vi "svc_Set SV Channel Info (variant).vi"(5 "channel description":string, 7 "channel name":string, 8 "error in (no error)":errorcluster, 10 "channel info":T1={"sensor sensitivity"=1000.0, "engineering units"=0, "dB reference"=1.0, "custom label"="EU", "weighting filter"=0, "pregain"=0.0} {"pregain" format="%.2f"; "weighting filter" items=["Linear", "A-weighting", "B-weighting", "C-weighting", "ITU-R 468-4", "Dolby", "CCITT", "C-message", "Wb", "Wc", "Wd", "We", "Wf", "Wh", "Wj", "Wk", "Wm", "AES17 20 kHz lowpass", "AES17 40 kHz lowpass", "AES17 20 kHz highpass", "AES17 40 kHz highpass"]; "dB reference" format="%^.1e"; "engineering units" items=["custom..."=0, "V"=1, "A"=21, "C"=30, "pC"=31, "s"=32, "-"=29, "Pa"=2, "N"=20, "g"=3, "m/s^2"=4, "m/s"=5, "m"=6, "mm/s"=12, "mm"=13, "micron/s"=14, "micron"=15, "in/s^2"=7, "in/s"=8, "in"=9, "mil/s"=10, "mil"=11, "rad/s^2"=16, "rad/s"=17, "rad"=18, "deg/s^2"=26, "deg/s"=27, "deg"=28, "RPM"=22, "cycle/s^2"=23, "Hz"=24, "cycle"=25, "strain"=19]; "sensor sensitivity" format="%#_5f"}, 11 "attributes":variant) -> (0 "error out":errorcluster, 3 "attributes":variant)   [LabVIEW 2017]
uses:
  <vilib>/addons/_NISVFA/_Shared subVIs/Controls/svc_Channel Info.ctl
  <vilib>/addons/_NISVFA/_Shared subVIs/Controls/svc_Engineering Units Text Ring.ctl
  <vilib>/addons/_NISVFA/_Shared subVIs/Controls/svc_Weighting Filter Text Ring.ctl
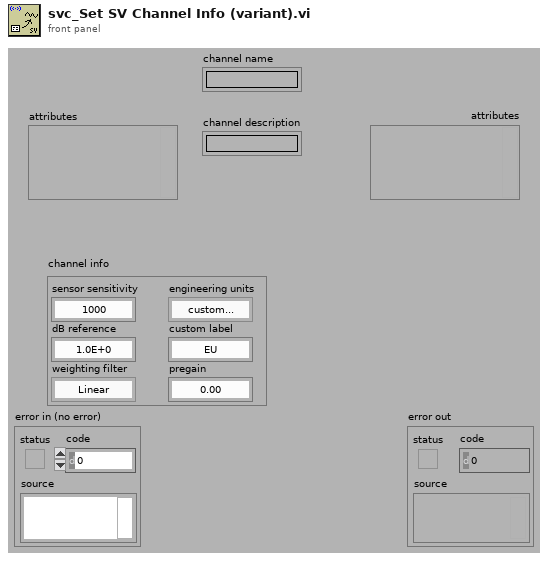
[diagram p1: front panel]
types:
  T1 = typedef "svc_Channel Info.ctl" = cluster{"sensor sensitivity":dbl, "engineering units":T2, "dB reference":dbl, "custom label":string, "weighting filter":T3, "pregain":dbl}
  T2 = typedef "svc_Engineering Units Text Ring.ctl" = u16
  T3 = typedef "svc_Weighting Filter Text Ring.ctl" = u16
  T4 = enum16{"custom...", "V", "Pa", "g", "m/s^2", "m/s", "m", "in/s^2", "in/s", "in", "mil/s", "mil", "mm/s", "mm", "micron/s", "micron", "rad/s^2", "rad/s", "rad", "strain", "N", "A", "rpm", "cycle/s^2", "Hz", "cycle", "deg/s^2", "deg/s", "deg", "Undefined", "C", "pC"}
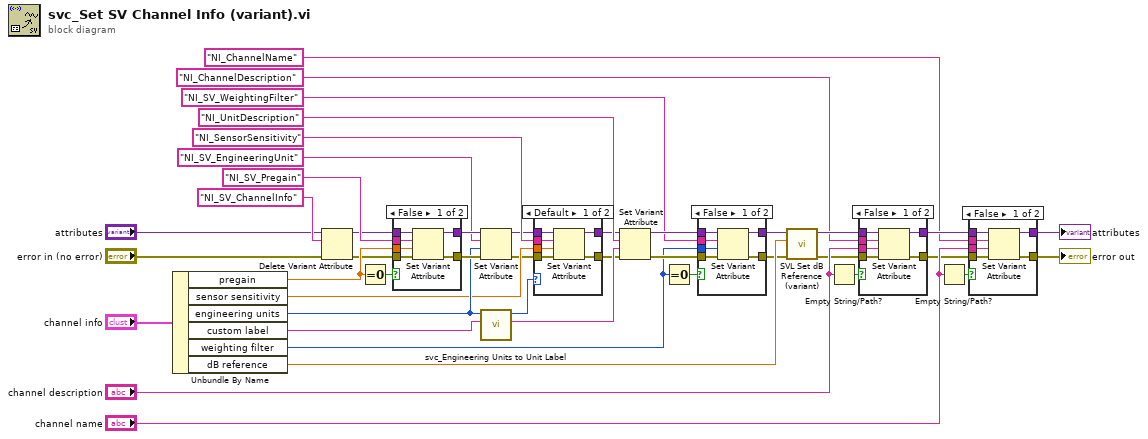
[diagram p0: block diagram]
diagram:
  n1 = Unbundle By Name("channel info") -> ("pregain"=w29:dbl, "sensor sensitivity"=w11:dbl, "engineering units"=w24:T2, "custom label"=w23:string, "weighting filter"=w14:T3, "dB reference"=w20:dbl)
  n2 = Delete Variant Attribute(4:"error in (no error)", 6:"NI_SV_ChannelInfo" ("name"), 7:"attributes") -> (0:w4:errorcluster, 3:w6:variant)  [unwired: 1 out]
  n3 = Equal To 0?(x=w29) -> (x = 0?=w30:bool)
  n4 = case shown="False" w30 {
    tunnel: w6 -> [w49 w51]
    tunnel: [w48 w51] -> w26
    tunnel: [w47 w50] -> w27
    tunnel: w4 -> [w46 w50]
    tunnel: w29 -> [w45 _]
    tunnel: "NI_SV_Pregain" ("name") -> [w44 _]
    frame False {
      n5 = Set Variant Attribute(Variant=w49, name=w44, value=w45, error in=w46) -> (Variant out=w48:variant, error out=w47:errorcluster)  [unwired: 1 out]
    }
    frame True {
    }
  }
  n6 = Set Variant Attribute(Variant=w26, name="NI_SV_EngineeringUnit", value=w24, error in=w27) -> (Variant out=w10:variant, error out=w9:errorcluster)  [unwired: 1 out]
  n7 = call <vilib>:"svc_Engineering Units to Unit Label.vi"("custom label"=w23, "engineering units"=w24) -> ("unit label"=w22:string, "engineering units enum"=w12:T4)  [unwired: 8 in]
  n8 = case shown="Default" w12 {
    tunnel: w10 -> [w57 w59]
    tunnel: [w56 w59] -> w8
    tunnel: [w55 w58] -> w7
    tunnel: w9 -> [w54 w58]
    tunnel: w11 -> [w53 _]
    tunnel: "NI_SensorSensitivity" ("name") -> [w52 _]
    frame Default {
      n9 = Set Variant Attribute(Variant=w57, name=w52, value=w53, error in=w54) -> (Variant out=w56:variant, error out=w55:errorcluster)  [unwired: 1 out]
    }
    frame "V" {
    }
  }
  n10 = Set Variant Attribute(Variant=w8, name="NI_UnitDescription", value=w22, error in=w7) -> (Variant out=w17:variant, error out=w16:errorcluster)  [unwired: 1 out]
  n11 = Equal To 0?(x=w14) -> (x = 0?=w13:bool)
  n12 = case shown="False" w13 {
    tunnel: w17 -> [w65 w67]
    tunnel: [w64 w67] -> w19
    tunnel: [w63 w66] -> w18
    tunnel: w16 -> [w62 w66]
    tunnel: w14 -> [w61 _]
    tunnel: "NI_SV_WeightingFilter" ("name") -> [w60 _]
    frame False {
      n13 = Set Variant Attribute(Variant=w65, name=w60, value=w61, error in=w62) -> (Variant out=w64:variant, error out=w63:errorcluster)  [unwired: 1 out]
    }
    frame True {
    }
  }
  n14 = call <vilib>:"SVL Set dB Reference (variant).vi"("error in (no error)"=w18, "dB reference [EU]"=w20, "attributes in"=w19) -> ("error out"=w36:errorcluster, "attributes out"=w39:variant)  [unwired: 7 in]
  n15 = Empty String/Path?(string/path="channel description") -> (empty?=w35:bool)
  n16 = case shown="False" w35 {
    tunnel: w39 -> [w73 w75]
    tunnel: [w72 w75] -> w38
    tunnel: [w71 w74] -> w37
    tunnel: w36 -> [w70 w74]
    tunnel: "channel description" -> [w69 _]
    tunnel: "NI_ChannelDescription" ("name") -> [w68 _]
    frame False {
      n17 = Set Variant Attribute(Variant=w73, name=w68, value=w69, error in=w70) -> (Variant out=w72:variant, error out=w71:errorcluster)  [unwired: 1 out]
    }
    frame True {
    }
  }
  n18 = Empty String/Path?(string/path="channel name") -> (empty?=w34:bool)
  n19 = case shown="False" w34 {
    tunnel: [w81 w83] -> w1
    tunnel: [w80 w82] -> w43
    tunnel: w38 -> [w79 w83]
    tunnel: w37 -> [w78 w82]
    tunnel: "channel name" -> [w77 _]
    tunnel: "NI_ChannelName" ("name") -> [w76 _]
    frame False {
      n20 = Set Variant Attribute(Variant=w79, name=w76, value=w77, error in=w78) -> (Variant out=w81:variant, error out=w80:errorcluster)  [unwired: 1 out]
    }
    frame True {
    }
  }
  "attributes" <- w1
  "error out" <- w43
